vi "Detect Single.vi"   [LabVIEW 2020, in "feature_detection.lvlib" / "QR Code Detector.lvclass"]
doc: "Detect a single QR Code in an Image. If multiple QR Codes are present then only one detection will be returned."
uses:
  QR Code Detector.lvclass
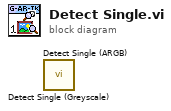
[diagram p0: block diagram]
diagram:
  n1 = call "Detect Single (Greyscale).vi"() -> ()  [unwired: 7 in, 5 out]
  n2 = call "Detect Single (ARGB).vi"() -> ()  [unwired: 7 in, 5 out]
